vi "zmq_geterr.vi"(1 "error in":errorcluster) -> (0 "type":T1)   [LabVIEW 2020, in "zeromq.lvlib"]
doc: "Checks an error cluster for errors originating from ZMQ, and returns an enum corresponding to which error it was."
uses:
  zeromq.lvlib
  error_type.ctl
panel:
  # "ØMQ"
  # "labview"
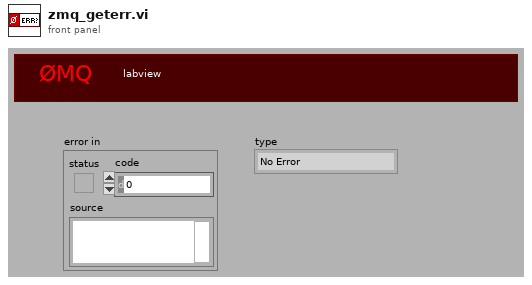
[diagram p1: front panel]
types:
  T1 = typedef "zeromq.lvlib/error_type.ctl" = enum16{"No Error", "EUNKNOWN", "ENOTSUP", "EPROTONOSUPPORT", "ENOBUFS", "ENETDOWN", "EADDRINUSE", "EADDRNOTAVAIL", "ECONNREFUSED", "EINPROGRESS", "ENOTSOCK", "EMSGSIZE", "EAFNOSUPPORT", "ENETUNREACH", "ECONNABORT", "ECONNRESET", "ENOTCONN", "ETIMEDOUT", "EHOSTUNREACH", "ENETRESET", "EBUSY", "EINVAL", "ENODEV", "EFAULT", "EINTR", "ENOENT", "ENOMEM", "EAGAIN", "EMFILE", "EFSM", "ENOCOMPATPROTO", "ETERM", "EMTHREAD", "Invalid"}
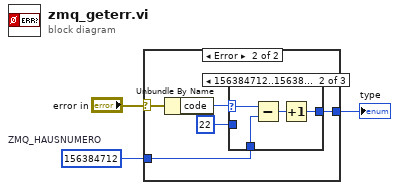
[diagram p0: block diagram]
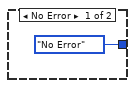
[diagram p2: hidden frame]
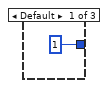
[diagram p3: hidden frame]
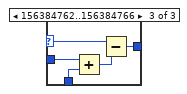
[diagram p4: hidden frame]
diagram:
  w1 = 156384712  # ZMQ_HAUSNUMERO
  n1 = case shown="Error" "error in" {
    selector: "error in" -> [_ w8]
    tunnel: [error_type."No Error" ("type") w9] -> w3
    tunnel: w1 -> [_ w6]
    frame No Error {
    }
    frame Error {
      n2 = Unbundle By Name(w8) -> ("code"=w7:i32)
      n3 = case shown="156384712..156384740" w7 {
        selector: w7 -> [_ w14 w18]
        tunnel: [1 w11 w19] -> w9
        tunnel: w6 -> [_ w12 w16]
        tunnel: 22 ("x") -> [_ _ w15]
        frame Default {
        }
        frame 156384712..156384740 {
          n4 = Subtract(x=w14, y=w12) -> (x-y=w13:i32)
          n5 = Increment(x=w13) -> (x+1=w11:i32)
        }
        frame 156384762..156384766 {
          n6 = Add(x=w15, y=w16) -> (x+y=w17:i32)
          n7 = Subtract(x=w18, y=w17) -> (x-y=w19:i32)
        }
      }
    }
  }
  "type" <- w3
